vi "test.vi"() -> ()   [LabVIEW 2009]
panel:
  in  "Gausswidth (px)":dbl
  out "Intensity Graph":dbl[][](graph)
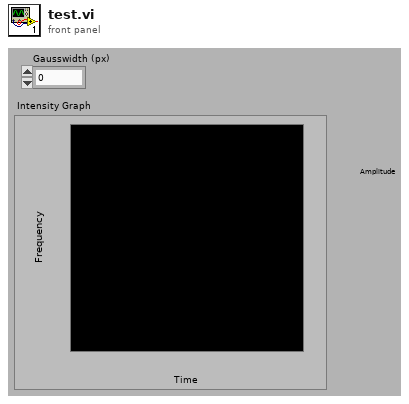
[diagram p1: front panel]
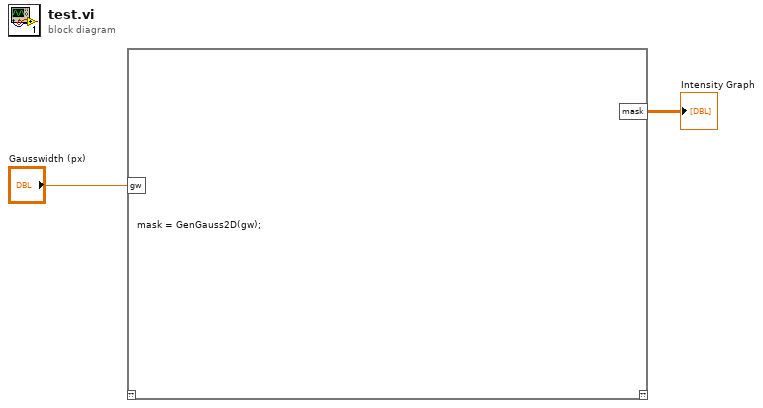
[diagram p0: block diagram]
diagram:
  n1 = script code="mask = GenGauss2D(gw);"("gw"="Gausswidth (px)") -> ("mask"=→"Intensity Graph":dbl[][])  [unwired: 1 in, 1 out]
